vi "NI VeriStand - Open UDP Channel Streaming Session.vi"(8 "error in (no error)":errorcluster, 10 "Channels":string[](array[string]), 11 "WorkspaceManager in":T1) -> (0 "error out":errorcluster, 2 "UDPChannelStreamSession out":T2, 3 "WorkspaceManager out":T1)   [LabVIEW 2020, in "NI_VS Workspace ExecutionAPI.lvlib"]
doc: "Opens a UDP channel streaming session. Use the Deploy UDP Channel Streaming Session VI to deploy the session and begin streaming channel data."
uses:
  <vilib>/NI VeriStand/Execution/Workspace/NI_VS Workspace ExecutionAPI.lvlib
  <vilib>/NI VeriStand/Execution/Workspace/WorkspaceAPI.ctl
  NationalInstruments.VeriStand.ClientAPI
  <vilib>/NI VeriStand/Execution/Workspace/UDPChannelStreamSession.ctl
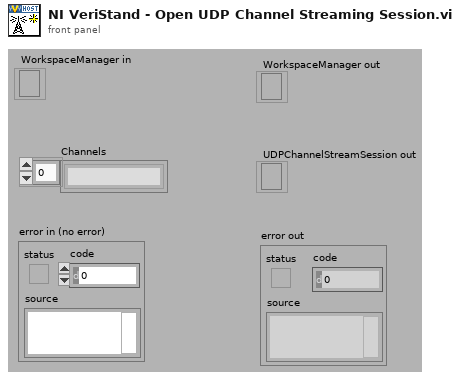
[diagram p1: front panel]
types:
  T1 = typedef "NI_VS Workspace ExecutionAPI.lvlib/WorkspaceAPI.ctl" = refnum<k24>
  T2 = typedef "NI_VS Workspace ExecutionAPI.lvlib/UDPChannelStreamSession.ctl" = refnum<k24>
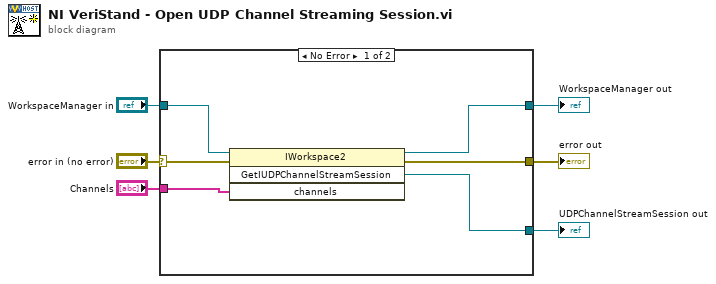
[diagram p0: block diagram]
diagram:
  n1 = case shown="No Error" "error in (no error)" {
    selector: "error in (no error)" -> [w12 w14]
    tunnel: [w8 w14] -> w6
    tunnel: "WorkspaceManager in" -> [w10 w13]
    tunnel: "Channels" -> [w11 _]
    tunnel: [w9 _] -> w2
    tunnel: [w7 w13] -> w1
    frame No Error {
      n2 = invoke class="IWorkspace2" method="GetIUDPChannelStreamSession"(reference=w10, error in=w12, "channels"=w11) -> (reference out=w7:T1, error out=w8:errorcluster, "GetIUDPChannelStreamSession"=w9:refnum<k24>)  [unwired: 1 in, 1 out]
    }
    frame Error {
    }
  }
  "error out" <- w6
  "UDPChannelStreamSession out" <- w2
  "WorkspaceManager out" <- w1
